vi "Register.vi"(8 "error in (no error)":errorcluster, 11 "logger in":refnum<class "Logger.lvclass">) -> (0 "error out":errorcluster)   [LabVIEW 2018, in "GLog.lvlib" / "Registry.lvlib"]
uses:
  Registry.lvlib
  api/logger_class/Logger.lvclass
  Registry Actions.ctl
  dependencies/Utilities/Utilities.lvlib
panel:
  # "Connector Pane"
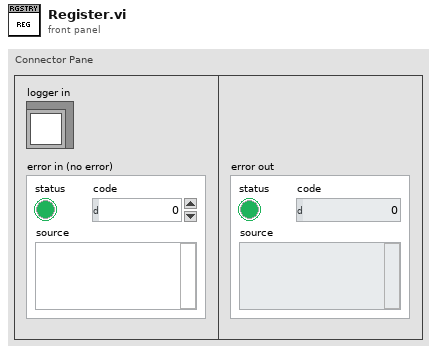
[diagram p1: front panel]
types:
  T1 = typedef "GLog.lvlib/Registry.lvlib/Registry Actions.ctl" = enum16{"Register", "Log", "Enable", "Enable All", "Disable", "Disable All", "Get Enable State", "Get Minimum Log Level", "Set Minimum Log Level", "Set All Minimum Log Level", "Get Logger Info", "Get All Logger Info", "List", "Unregister", "Unregister All", "Shutdown"}
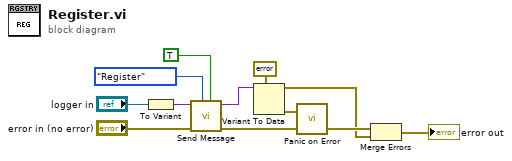
[diagram p0: block diagram]
diagram:
  n1 = To Variant(anything="logger in") -> (Variant=w8:variant)
  n2 = call "Send Message.vi"("return data? (F)"=TRUE, "action"=Registry_Actions."Register", "error in (no error)"="error in (no error)", "send data"=w8) -> ("error out"=w11:errorcluster, "return data"=w6:variant)  [unwired: 6 in]
  n3 = Variant To Data(type=errorcluster {"status"=FALSE, "code"=0, "source"=""} ("error in (no error)"), Variant=w6) -> (data=w2:errorcluster, error out=w4:errorcluster)  [unwired: 1 in]
  n4 = call "Panic on Error.vi"("error in (no error)"=w4) -> ()  [unwired: 3 in]
  n5 = Merge Errors(w11, w2) -> (→"error out":errorcluster)
